vi "Device Identity.vi"(8 "error in (no error)":errorcluster, 11 "Session in":refnum<class "Session.lvclass">) -> (0 "error out":errorcluster, 2 "Identity":T1, 3 "Session out":refnum<class "Session.lvclass">)   [LabVIEW 2024, in "CTI.lvlib" / "Session.lvclass"]
doc: "Queries the device firmware for the device's identity which can be used to check for compatibility, handle differences between different device types, and differentiate between different devices of the same type. When possible, every device of the same Model will return a unique Serial Number."
uses:
  Session.lvclass
  Identity.ctl
  DeviceComms/DeviceComms.lvclass
  CTI.lvlib
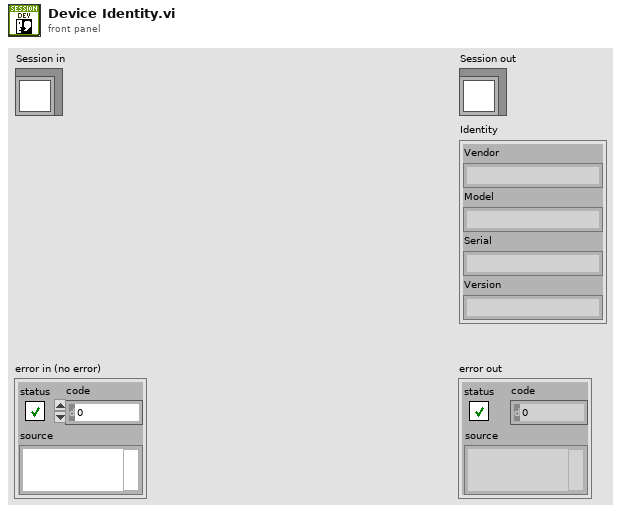
[diagram p1: front panel]
types:
  T1 = typedef "CTI.lvlib/Identity.ctl" = cluster{"Vendor":string, "Model":string, "Serial":string, "Version":string}
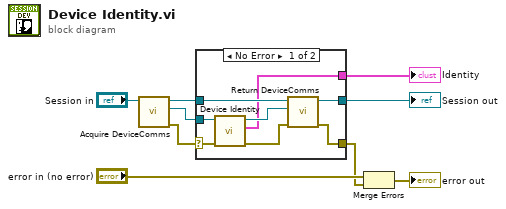
[diagram p0: block diagram]
diagram:
  n1 = call "Acquire DeviceComms.vi"("Session in"="Session in") -> ("error out"=w6:errorcluster, "DeviceComms"=w5:refnum<class "DeviceComms.lvclass">, "Session out"=w7:refnum<class "Session.lvclass">)  [unwired: 8 in]
  n2 = case shown="No Error" w6 {
    selector: w6 -> [w16 w19]
    tunnel: w7 -> [w15 w18]
    tunnel: w5 -> [w17 _]
    tunnel: [w10 _] -> w4
    tunnel: [w12 w18] -> w3
    tunnel: [w11 w19] -> w1
    frame No Error {
      n3 = call-dynamic "Device Identity.vi"("error in (no error)"=w16, "DeviceComms in"=w17) -> ("error out"=w13:errorcluster, "Identity"=w10:T1, "DeviceComms out"=w14:refnum<class "DeviceComms.lvclass">)  [unwired: 7 in]
      n4 = call "Return DeviceComms.vi"("error in (no error)"=w13, "DeviceComms"=w14, "Session in"=w15) -> ("error out"=w11:errorcluster, "Session out"=w12:refnum<class "Session.lvclass">)  [unwired: 7 in]
    }
    frame Error {
    }
  }
  "Session out" <- w3
  "Identity" <- w4
  n5 = Merge Errors("error in (no error)", w1) -> (→"error out":errorcluster)
